vi "createFile.vi"() -> ()   [LabVIEW 2019]
uses:
  <vilib>/Utility/file.llb/Write Delimited Spreadsheet (DBL).vi
panel:
  in  "2D data":dbl[][](array[numeric])
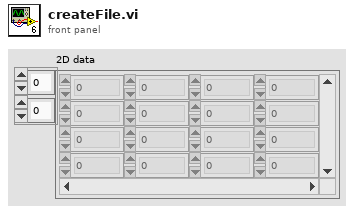
[diagram p1: front panel]
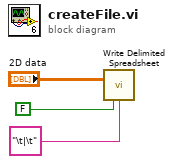
[diagram p0: block diagram]
diagram:
  n1 = call-poly <vilib>:"Write Delimited Spreadsheet.vi"("2D data"="2D data", "transpose? (no:F)"=FALSE, "delimiter (\\t)"="\t|\t" ("delimiter (\\t)")) -> ()  [unwired: 11 in, 2 out]
